vi "String to TimerDays Array.vi"(8 "error in (no error)":errorcluster, 11 "Timer Days":string) -> (0 "error out":errorcluster, 3 "Start/End Days":T1(array[ring]))   [LabVIEW 2016, in "Environment Chamber.lvlib" / "Climatic Chamber.lvlib"]
uses:
  Climatic Chamber.lvlib
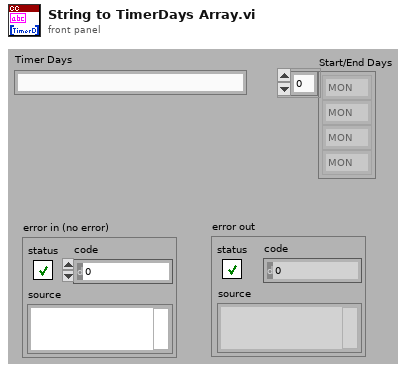
[diagram p1: front panel]
types:
  T1 = enum16{"MON", "TUE", "WED", "THU", "FRI", "SAT", "SUN"}[]
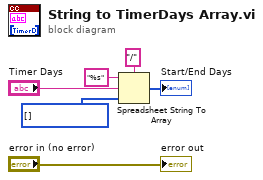
[diagram p0: block diagram]
diagram:
  w3 = T1 [] items=["MON", "TUE", "WED", "THU", "FRI", "SAT", "SUN"] ("Start/End Days")
  n1 = Spreadsheet String To Array(delimiter (Tab)="/", format string="%s", spreadsheet string="Timer Days", array type (2D Dbl)=w3) -> (array=→"Start/End Days":T1)
  "error out" <- "error in (no error)"
